vi "Resolve (DBL).vi"(8 "error in (no error)":errorcluster, 10 "Element":refnum<class "Config Element.lvclass">, 11 "Sequence Constants in":refnum<class "Sequence Constants.lvclass">) -> (0 "error out":errorcluster, 2 "DBL Value":dbl, 3 "Sequence Constants out":refnum<class "Sequence Constants.lvclass">)   [LabVIEW 2020, in "VolatusSeqConfig.lvlib" / "Sequence Constants.lvclass"]
uses:
  Sequence Constants.lvclass
  lv-cdm/CDM-Config/Config Element/Config Element.lvclass
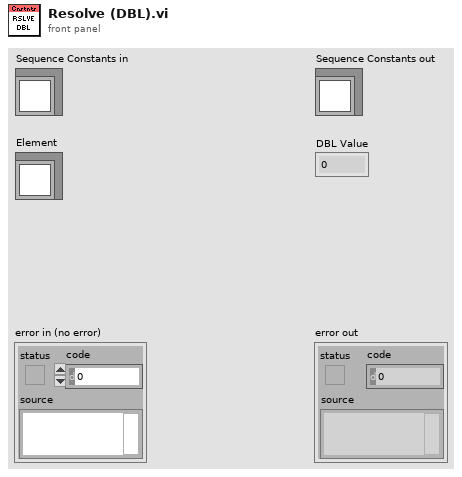
[diagram p1: front panel]
types:
  T1 = typedef "CDM-Config.lvlib/Value Type.ctl" = enum16{"String", "Number", "Bool", "Object", "Array"}
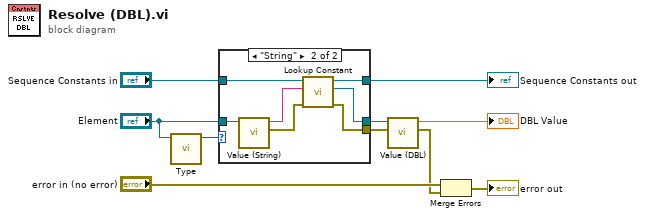
[diagram p0: block diagram]
diagram:
  n1 = call "Type.vi"("Config Element in"="Element") -> ("Value Type"=w9:T1)  [unwired: 9 in, 1 out]
  n2 = case shown="\"String\"" w9 {
    tunnel: "Element" -> [w11 w19]
    tunnel: "Sequence Constants in" -> [w12 w18]
    tunnel: [w12 w14] -> w7
    tunnel: [_ w16] -> w3
    tunnel: [w11 w15] -> w4
    frame Default {
    }
    frame "String" {
      n3 = call "Value (String).vi"("Config Element in"=w19) -> ("error out"=w13:errorcluster, "String Value"=w17:string)  [unwired: 9 in]
      n4 = call "Lookup Constant.vi"("error in (no error)"=w13, "Constant Name"=w17, "Sequence Constants in"=w18) -> ("error out"=w16:errorcluster, "Element"=w15:refnum<class "Config Element.lvclass">, "Sequence Constants out"=w14:refnum<class "Sequence Constants.lvclass">)  [unwired: 6 in]
    }
  }
  "Sequence Constants out" <- w7
  n5 = call "Value (DBL).vi"("error in (no error)"=w3, "Config Element in"=w4) -> ("error out"=w2:errorcluster, "DBL Value"=→"DBL Value":dbl)  [unwired: 8 in]
  n6 = Merge Errors("error in (no error)", w2) -> (→"error out":errorcluster)
